vi "collectAI_tt_V2.vi"   [LabVIEW 2015]
uses:
  <vilib>/DAQmx/read.llb/DAQmx Read (Analog 2D I16 NChan NSamp).vi
  <vilib>/DAQmx/miscellaneous.llb/DAQmx Fill In Error Info.vi
types:
  T1 = typedef "LVRectTypeDef.ctl" = cluster{"Left":i16, "Top":i16, "Right":i16, "Bottom":i16}
  T2 = cluster{"Xpixels":i32, "Vxminref":dbl, "Vxmaxref":dbl, "P":dbl, "Ypixels":i32, "Vyminref":dbl, "Vymaxref":dbl, "srate":sgl, "sAOxy":i32, "timeout":dbl, "type":string, "date":string, "time":string, "Colormap":u16, "Drawing Mode":u16, "Scanning Mode":u16, "square pixels":bool, "square matrix":bool, "Xpixels Img":i32, "Vx-min Img":dbl, "VX-max Img":dbl, "Ypixels Img":i32, "Vy-min Img":dbl, "Vy-max Img ":dbl, "Angle Img":dbl, "autoshutter":bool, "finite":bool, "cont":bool, "wavdet":bool, "measpoints":i32, "avpp":i32, "bufferAO":i32, "bufferAI":i32, "starttick":u32, "waveform":path, "Vx-ref":dbl, "Vy-ref":dbl, "refreshrate":dbl, "refreshbuffer":i32, "tt_cycles":i32, "motorref":refnum<k7>, "mirrorswitch":refnum<k7>, "sample mode":i32, "maxbufferAI":i32, "srateAODO":sgl, "bin":sgl, "Pel":sgl, "Angle draw":dbl, "srate Img":sgl, "ROIimg_plotbounds":T1, "auto OD":bool, "ODfilt":u16, "aAI":i32[], "aCI":i32[], "aAO":u32[], "aDO":u32[], "refwfsize":dbl, "Lifetime":bool, "Vz-Img":dbl, "Vz-ref":dbl, "Vz-reset":dbl, "AIoverride":bool, "aAS":u32[], "XYZstart":dbl[], "External 100KHz Clock?":bool}
  T3 = cluster{" AI":refnum<k21>, "E_AI":errorcluster, "header":dbl[]}
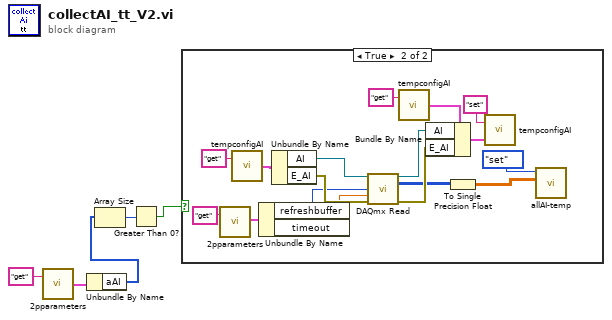
[diagram p0: block diagram]
diagram:
  n1 = call "2pparameters.vi"("command"="get") -> ("params out"=w4:T2)  [unwired: 1 in]
  n2 = Unbundle By Name(w4) -> ("aAI"=w3:i32[])
  n3 = Array Size(array=w3) -> (size(s)=w2:i32)
  n4 = Greater Than 0?(x=w2) -> (x > 0?=w1:bool)
  n5 = case shown="True" w1 {
    frame False {
    }
    frame True {
      n6 = call "2pparameters.vi"("command"="get") -> ("params out"=w9:T2)  [unwired: 1 in]
      n7 = call "tempconfigAI.vi"("command"="get") -> ("Temp Config out"=w19:T3)  [unwired: 1 in]
      n8 = Unbundle By Name(w9) -> ("refreshbuffer"=w12:i32, "timeout"=w11:dbl)
      n9 = Unbundle By Name(w19) -> ("AI"=w18:refnum<k21>, "E_AI"=w17:errorcluster)
      n10 = call-poly <vilib>:"DAQmx Read.vi"("task/channels in"=w18, "number of samples per channel"=w12, "timeout"=w11, "error in"=w17) -> ("task out"=w13:refnum<k21>, "data"=w6:i16[][], "error out"=w22:errorcluster)  [unwired: 9 in]
      n11 = call "tempconfigAI.vi"("command"="get") -> ("Temp Config out"=w14:T3)  [unwired: 1 in]
      n12 = Bundle By Name(cluster=w14, "AI"=w13, "E_AI"=w22) -> (w21:T3)
      n13 = To Single Precision Float(number=w6) -> (single precision float=w8:sgl[][])
      n14 = call "tempconfigAI.vi"("Temp Config in"=w21, "command"="set") -> ()  [unwired: 1 out]
      n15 = call "allAI-temp.vi"("array in"=w8, "command"=enum16{"get", "set", "clear", "append"}."set") -> ()  [unwired: 2 in, 2 out]
    }
  }
